vi "Launch Deferred Timeout Notifier.vi"(8 "error in (no error)":errorcluster, 9 "Timeout [ms]":i32=1000, 10 "Timeout Action":T1, 11 "Message Cycle Notifier":refnum<notifier>) -> (0 "error out":errorcluster, 2 "Timeout Notifier":refnum<notifier>)   [LabVIEW 2020, in "MVA Framework.lvlib" / "MessageCycle.lvclass"]
doc: "等待指定的时间量，然后向参与者发送指定次数的消息。"
uses:
  MessageCycle.lvclass
  Message Cycle Notifications.ctl
  Timeout Notifications.ctl
  Timeout Notifier Core.vi
  MessageCycle.lvclass/MessageCycle.ctl
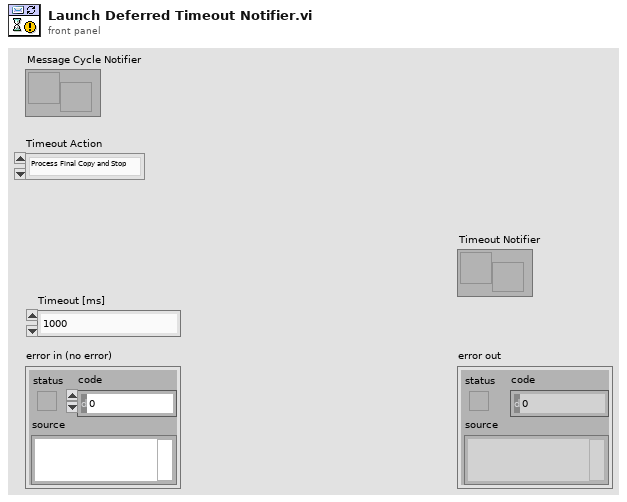
[diagram p1: front panel]
types:
  T1 = typedef "MVA Framework.lvlib/MessageCycle.lvclass/Message Cycle Notifications.ctl" = enum16{"Process Final Copy and Stop", "Stop Immediately", "Substitute Last Message and Stop"}
  T2 = typedef "MVA Framework.lvlib/MessageCycle.lvclass/Timeout Notifications.ctl" = enum16{"Cancel Timeout", "Force Timeout"}
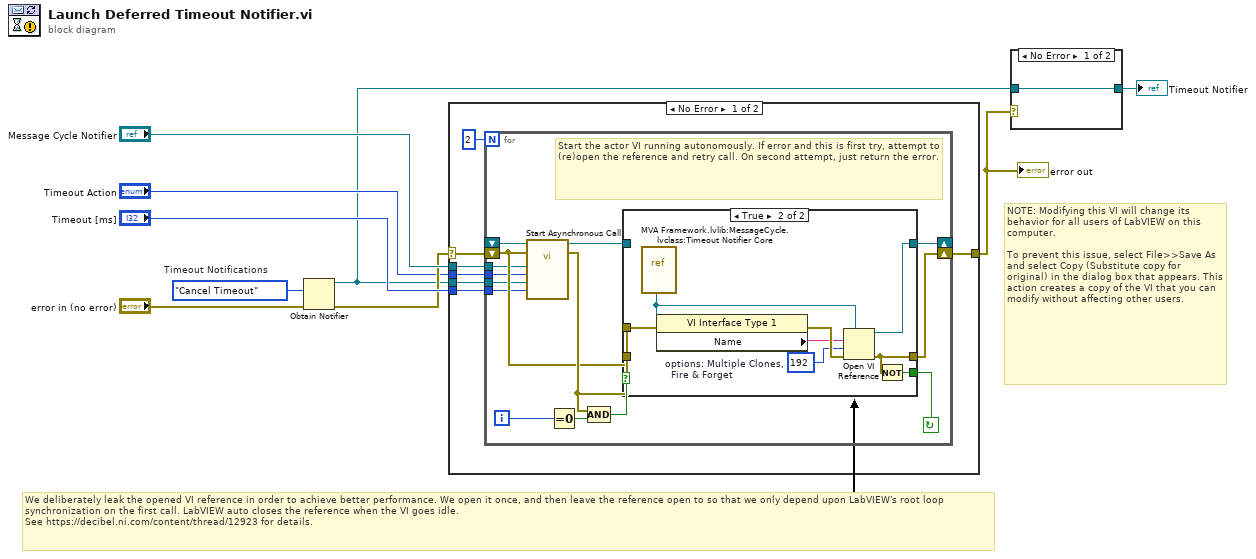
[diagram p0: block diagram]
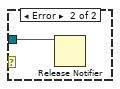
[diagram p4: hidden frame]
diagram:
  w9 = Timeout_Notifications."Cancel Timeout"  # Timeout Notifications
  # "We deliberately leak the opened VI reference in order to achieve better performance. We open it once, and then leave the reference open to so that we only depend upon LabVIEW's root loop synchronization on the first call. LabVIEW auto closes the reference when the VI goes idle. \nSee https://decibel.ni.com/content/thread/12923 for details."
  # "NOTE: Modifying this VI will change its behavior for all users of LabVIEW on this computer.\n\nTo prevent this issue, select File>>Save As and select Copy (Substitute copy for original) in the dialog box that appears. This action creates a copy of the VI that you can modify without affecting other users."
  n1 = Obtain Notifier(notification data type=w9, error in (no error)="error in (no error)") -> (notifier out=w1:refnum<notifier>, error out=w3:errorcluster)  [unwired: 2 in, 1 out]
  n2 = case shown="No Error" w3 {
    selector: w3 -> [w14 w41]
    tunnel: [w15 w41] -> w4
    tunnel: "Timeout [ms]" -> [w13 _]
    tunnel: "Timeout Action" -> [w12 _]
    tunnel: w1 -> [w11 _]
    tunnel: "Message Cycle Notifier" -> [w10 _]
    frame No Error {
      n3 = for {
        N: 2 -> [_]
        shift-right: [w30] -> _
        shift-left: _ -> [w23]
        shift-right: [w29] -> w15
        shift-left: w14 -> [w24]
        tunnel: w13 -> [w21]
        tunnel: w12 -> [w20]
        tunnel: w11 -> [w19]
        tunnel: w10 -> [w18]
        i -> [w26]
        stop <- w17 continue-if-true
        # "Start the actor VI running autonomously. If error and this is first try, attempt to (re)open the reference and retry call. On second attempt, just return the error."
        n4 = call-by-ref "Start Asynchronous Call"(reference=w23, error in=w24, "Time To Wait"=w21, "Timeout Notifier"=w19, "Timeout Action"=w20, "Message Cycle Notifier"=w18) -> (reference out=w22:refnum<vi>, error out=w25:errorcluster)  [unwired: 8 in]
        n5 = Equal To 0?(x=w26) -> (x = 0?=w27:bool)
        n6 = Compound Arithmetic op=AND(w25, w27) -> (w28:bool)
        n7 = case shown="True" w28 {
          tunnel: [w32 w37] -> w30
          tunnel: [w31 w35] -> w29
          tunnel: w22 -> [w32 _]
          tunnel: w25 -> [w31 _]
          tunnel: [_ w36] -> w17
          tunnel: w24 -> [_ w34]
          frame False {
          }
          frame True {
            w38 = 192  # options: Multiple Clones,   Fire & Forget
            n8 = vi-ref "MVA Framework.lvlib:MessageCycle.lvclass:Timeout Notifier Core.vi"() -> (w33:refnum<vi>)
            n9 = property class="VI Interface Type 1"(reference=w33, error in=w34) -> (error out=w40:errorcluster, "Name"=w39:string)  [unwired: 1 out]
            n10 = Open VI Reference(type specifier VI Refnum (for type only)=w33, vi path=w39, options=w38, error in (no error)=w40) -> (vi reference=w37:refnum<vi>, error out=w35:errorcluster)  [unwired: 2 in]
            n11 = Not(x=w35) -> (.not. x?=w36:bool)
          }
        }
      }
    }
    frame Error {
    }
  }
  "error out" <- w4
  n12 = case shown="No Error" w4 {
    tunnel: [w42 _] -> w7
    tunnel: w1 -> [w42 w43]
    frame No Error {
    }
    frame Error {
      n13 = Release Notifier(notifier=w43) -> ()  [unwired: 2 in, 3 out]
    }
  }
  "Timeout Notifier" <- w7
